vi "StartUp Sequence Open Loop Rev 1.0.vi"() -> ()   [LabVIEW 2017]
panel:
  out "Error Out":errorcluster
  in  "Error In":errorcluster
  in  "ECU COM Port":refnum<visa-resource-name>
  out "Turbine RPM":dbl
  out "Turbine Temp":dbl format="%.1f"
  out "Pump Voltage":dbl format="%.1f"
  out "Throttle Position":dbl format="%.1f"
  out "Turbine State":string
  in  "Strt Sqnc":bool
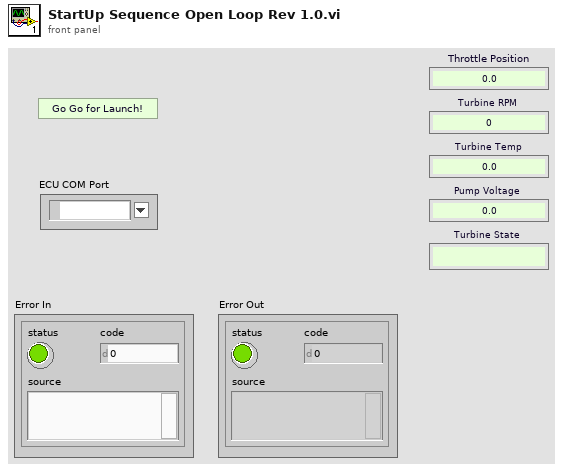
[diagram p1: front panel]
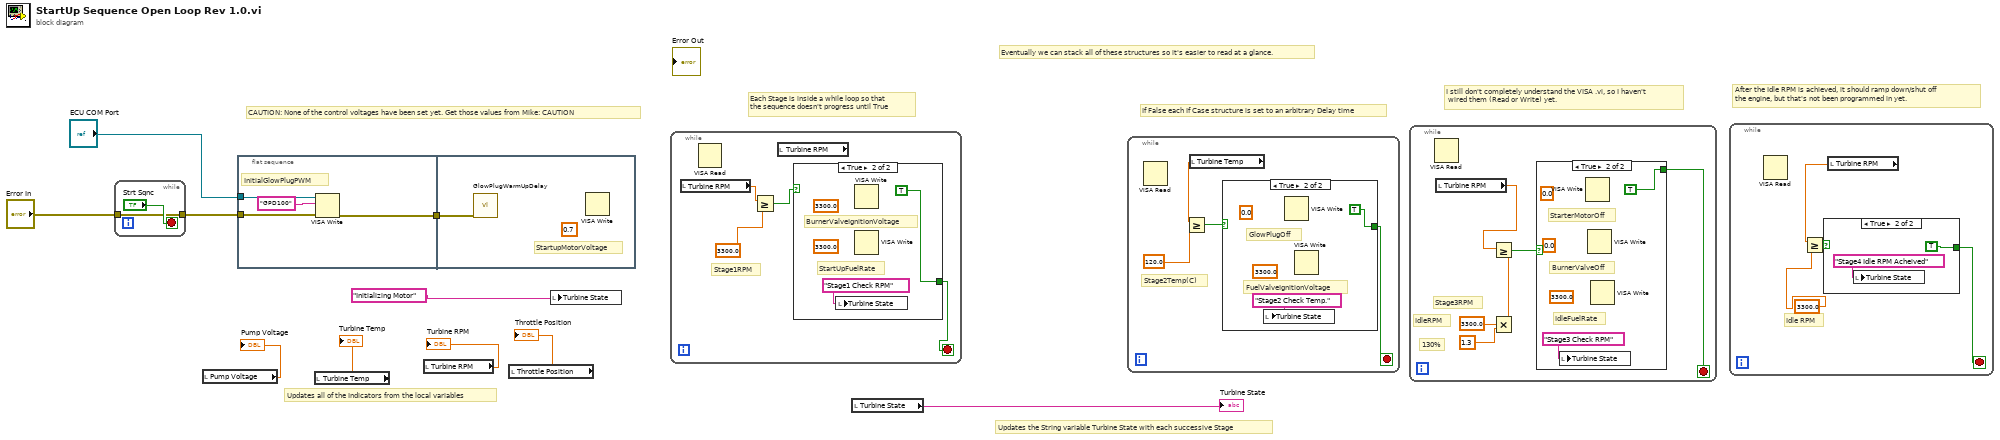
[diagram p0: block diagram]
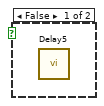
[diagram p2: hidden frame]
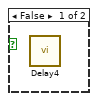
[diagram p3: hidden frame]
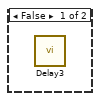
[diagram p4: hidden frame]
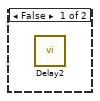
[diagram p5: hidden frame]
diagram:
  # "Eventually we can stack all of these structures so it's easier to read at a glance."
  # "Updates all of the Indicators from the local variables"
  # "After the Idle RPM is achieved, it should ramp down/shut off\nthe engine, but that's not been programmed in yet."
  # "I still don't completely understand the VISA .vi, so I haven't\n wired them (Read or Write) yet."
  # "CAUTION: None of the control voltages have been set yet. Get those values from Mike: CAUTION"
  # "Updates the String variable Turbine State with each successive Stage"
  # "If False each If Case structure is set to an arbitrary Delay time"
  # "Each Stage is inside a while loop so that \nthe sequence doesn't progress until True"
  n1 = while {
    tunnel: "Error In" -> [w11]
    tunnel: [w11] -> w3
    stop <- "Strt Sqnc" stop-if-true
  }
  n2 = local read "Pump Voltage"() -> (→"Pump Voltage":dbl)
  n3 = flat-sequence {
    tunnel: w3 -> [w15]
    tunnel: "ECU COM Port" -> [w16]
    tunnel: [w14] -> w1
    tunnel: w1 -> [w17]
    frame #0 {
      # "InitialGlowPlugPWM"
      n4 = VISA Write(VISA resource name=w16, write buffer="GPD100", error in (no error)=w15) -> (error out=w14:errorcluster)  [unwired: 2 out]
    }
    frame #1 {
      (unwired) 0.7
      # "StartupMotorVoltage"
      n5 = call "GlowPlugWarmUpDelay"("error in (no error)"=w17) -> ()  [unwired: 10 in, 1 out]
      n6 = VISA Write() -> ()  [unwired: 3 in, 3 out]
    }
  }
  n7 = local read "Turbine Temp"() -> (→"Turbine Temp":dbl)
  n8 = local read "Turbine RPM"() -> (→"Turbine RPM":dbl)
  n9 = local read "Throttle Position"() -> (→"Throttle Position":dbl)
  n10 = local write "Turbine State"("Initializing Motor") -> ()
  n11 = while {
    stop <- w20 stop-if-true
    # "Stage1RPM"
    n12 = local read "Turbine RPM"() -> (w19:dbl)
    n13 = VISA Read() -> ()  [unwired: 3 in, 4 out]
    n14 = Greater Or Equal?(x=w19, y=3300.0) -> (x >= y?=w22:bool)
    n15 = local read "Turbine RPM"() -> (w18:dbl)
    n16 = case shown="True" w22 {
      tunnel: [_ w23] -> _
      tunnel: [_ w23] -> w20
      frame False {
        n17 = call "Delay2"() -> ()  [unwired: 11 in, 1 out]
      }
      frame True {
        (unwired) 3300.0
        (unwired) 3300.0
        w23 = TRUE
        # "StartUpFuelRate"
        # "BurnerValveIgnitionVoltage"
        n18 = local write "Turbine State"("Stage1 Check RPM") -> ()
        n19 = VISA Write() -> ()  [unwired: 3 in, 3 out]
        n20 = VISA Write() -> ()  [unwired: 3 in, 3 out]
      }
    }
  }
  n21 = local read "Turbine State"() -> (→"Turbine State":string)
  n22 = while {
    stop <- w26 stop-if-true
    # "Stage2Temp(C)"
    n23 = VISA Read() -> ()  [unwired: 3 in, 4 out]
    n24 = local read "Turbine Temp"() -> (w25:dbl)
    n25 = Greater Or Equal?(x=w25, y=120.0) -> (x >= y?=w28:bool)
    n26 = case shown="True" w28 {
      tunnel: [_ TRUE] -> w26
      frame False {
        n27 = call "Delay3"() -> ()  [unwired: 11 in, 1 out]
      }
      frame True {
        (unwired) 3300.0
        (unwired) 0.0
        # "FuelValveIgnitionVoltage"
        # "GlowPlugOff"
        n28 = local write "Turbine State"("Stage2 Check Temp.") -> ()
        n29 = VISA Write() -> ()  [unwired: 3 in, 3 out]
        n30 = VISA Write() -> ()  [unwired: 3 in, 3 out]
      }
    }
  }
  n31 = while {
    stop <- w32 stop-if-true
    # "Stage3RPM"
    # "130%"
    # "IdleRPM"
    n32 = VISA Read() -> ()  [unwired: 3 in, 4 out]
    n33 = local read "Turbine RPM"() -> (w31:dbl)
    n34 = Multiply(x=3300.0, y=1.3) -> (x*y=w33:dbl)
    n35 = Greater Or Equal?(x=w31, y=w33) -> (x >= y?=w36:bool)
    n36 = case shown="True" w36 {
      tunnel: [_ TRUE] -> w32
      frame False {
        n37 = call "Delay4"() -> ()  [unwired: 11 in, 1 out]
      }
      frame True {
        (unwired) 3300.0
        (unwired) 0.0
        (unwired) 0.0
        # "IdleFuelRate"
        # "BurnerValveOff"
        # "StarterMotorOff"
        n38 = local write "Turbine State"("Stage3 Check RPM") -> ()
        n39 = VISA Write() -> ()  [unwired: 3 in, 3 out]
        n40 = VISA Write() -> ()  [unwired: 3 in, 3 out]
        n41 = VISA Write() -> ()  [unwired: 3 in, 3 out]
      }
    }
  }
  n42 = while {
    stop <- w40 stop-if-true
    # "Idle RPM"
    n43 = VISA Read() -> ()  [unwired: 3 in, 4 out]
    n44 = local read "Turbine RPM"() -> (w39:dbl)
    n45 = Greater Or Equal?(x=w39, y=3300.0) -> (x >= y?=w42:bool)
    n46 = case shown="True" w42 {
      tunnel: [_ TRUE] -> w40
      frame False {
        n47 = call "Delay5"() -> ()  [unwired: 11 in, 1 out]
      }
      frame True {
        n48 = local write "Turbine State"("Stage4 Idle RPM Acheived") -> ()
      }
    }
  }
